vi "DecodeBarcode.vi"   [LabVIEW 2026]
uses:
  vision_core_c/bin/barcode_decode.dll
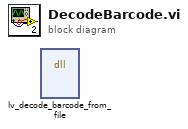
[diagram p0: block diagram]
diagram:
  n1 = dll-call lib="D:/git_proj/LabC-Vision/vision_core_c/bin/barcode_decode.dll" fn="lv_decode_barcode_from_file"() -> ()  [unwired: 10 in, 2 out]
